vi "TestEvaluator.vi"() -> ()   [LabVIEW 2023]
uses:
  Objectives.ctl
  Zone_class/Zone.lvclass
  Evaluator.lvclass
  Field_class/Field.lvclass
  Ball_class/Ball.lvclass
  C:/Users/ebert/Documents/codes/SSL/repo/SSL_AI/Object_class/Object.lvclass
  Object_class/Object.lvclass/Object.ctl
  Object_class/Object.lvclass
panel:
  in  "objectiveVector":T1[](array[typedef])
  out "field_width":i32
  out "field_length":i32
  in  "position(x,y)":dbl[](array[numeric])=[0.0, 0.0]
  out "evalMatrix":dbl[][](array[numeric])
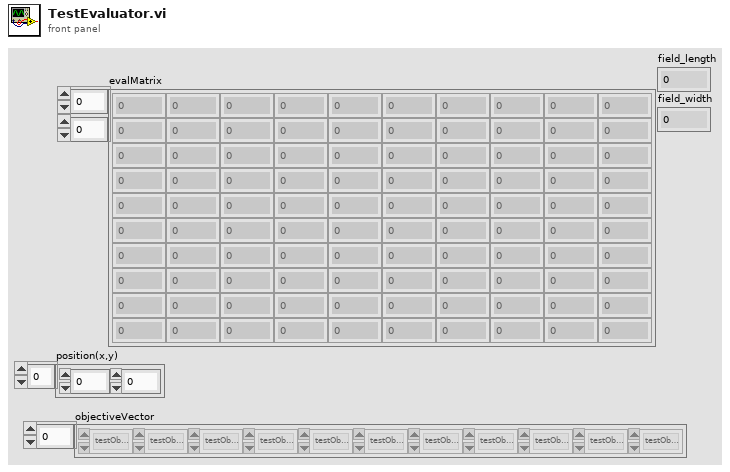
[diagram p1: front panel]
types:
  T1 = typedef "Evaluator.lvclass/Objectives.ctl" = enum16{"testObjective"}
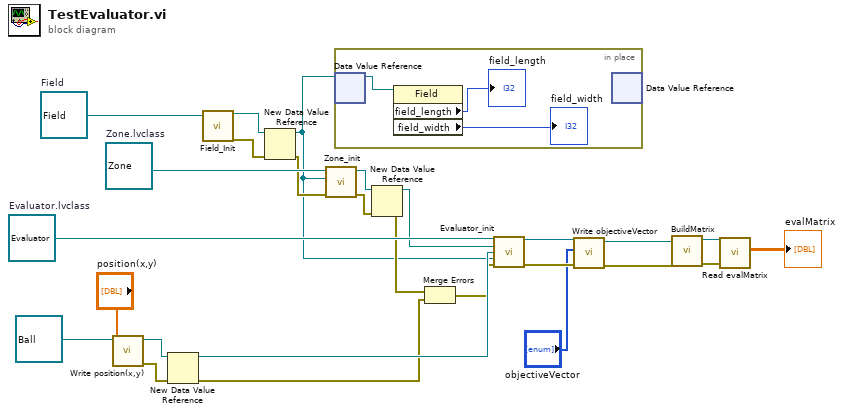
[diagram p0: block diagram]
diagram:
  w26 = refnum<class "Field.lvclass"> refnum  # Field
  w17 = refnum<class "Evaluator.lvclass"> refnum  # Evaluator.lvclass
  w25 = refnum<class "Zone.lvclass"> refnum  # Zone.lvclass
  n1 = call "Write position(x,y).vi"("position(x,y)"="position(x,y)", "Object in"=refnum<class "Ball.lvclass"> refnum ("Ball")) -> ("error out"=w11:errorcluster, "Object out"=w18:refnum<class "Ball.lvclass">)  [unwired: 8 in]
  n2 = New Data Value Reference(data value=w18, error in=w11) -> (data value reference=w15:refnum<data-value>, error out=w9:errorcluster)
  n3 = call "Field_Init.vi"("object in"=w26) -> ("object out"=w24:refnum<class "Field.lvclass">, "error out"=w14:errorcluster)  [unwired: 17 in]
  n4 = New Data Value Reference(data value=w24, error in=w14) -> (data value reference=w6:refnum<data-value>, error out=w13:errorcluster)
  n5 = call "Zone_init.vi"("error in (no error)"=w13, "FieldDVR"=w6, "Zone in"=w25) -> ("error out"=w12:errorcluster, "Zone out"=w23:refnum<class "Zone.lvclass">)  [unwired: 7 in]
  n6 = in-place {
    n7 = in-place-dvr #1(w6) -> (w27:refnum<class "Field.lvclass">)  [unwired: 1 out]
    n8 = property class="Field"(reference=w27) -> ("field_length"=→"field_length":i32, "field_width"=→"field_width":i32)  [unwired: 1 in, 2 out]
    n9 = in-place-dvr #1() -> ()  [unwired: 1 in, 2 out]
  }
  n10 = New Data Value Reference(data value=w23, error in=w12) -> (data value reference=w16:refnum<data-value>, error out=w10:errorcluster)
  n11 = Merge Errors(w10, w9) -> (w8:errorcluster)
  n12 = call-dynamic "Evaluator_init.vi"("Evaluator in"=w17, "ZoneDVR"=w16, "BallDVR"=w15, "FieldDVR"=w6, "error in (no error)"=w8) -> ("Evaluator out"=w5:refnum<class "Evaluator.lvclass">, "error out"=w3:errorcluster)  [unwired: 9 in]
  n13 = call-dynamic "Write objectiveVector.vi"("error in (no error)"=w3, "objectiveVector"="objectiveVector", "Evaluator in"=w5) -> ("error out"=w2:errorcluster, "Evaluator out"=w4:refnum<class "Evaluator.lvclass">)  [unwired: 7 in]
  n14 = call-dynamic "BuildMatrix.vi"("error in (no error)"=w2, "Evaluator in"=w4) -> ("error out"=w7:errorcluster, "Evaluator out"=w22:refnum<class "Evaluator.lvclass">)  [unwired: 8 in]
  n15 = call-dynamic "Read evalMatrix.vi"("error in (no error)"=w7, "Evaluator in"=w22) -> ("evalMatrix"=→"evalMatrix":dbl[][])  [unwired: 7 in, 2 out]
